vi "Read Transport.vi"(11 "ISubscriptionPolicy in":refnum<class "BasicSubscription.lvclass">) -> (2 "Transport":refnum<class "ITransport.lvclass">)   [LabVIEW 2015]
uses:
  BasicSubscription.lvclass
  IMediator/ITransport/ITransport.lvclass
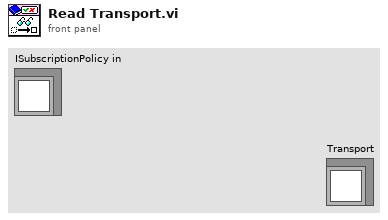
[diagram p1: front panel]
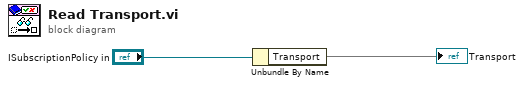
[diagram p0: block diagram]
diagram:
  n1 = Unbundle By Name("ISubscriptionPolicy in") -> ("Transport"=→"Transport")
